vi "Get Relay Position.vi"(8 "error in (no error)":errorcluster, 10 "relay name":string, 11 "SLSC Switch in":refnum<class "SLSC Switch.lvclass">) -> (0 "error out":errorcluster, 2 "position":T1=10 items=["Open"=10, "Closed"=11], 3 "SLSC Switch out":refnum<class "SLSC Switch.lvclass">)   [LabVIEW 2015, in "SLSC Switch.lvlib" / "SLSC Switch.lvclass"]
doc: "Returns the relay position for the relay specified in relay name."
uses:
  SLSC Switch.lvclass
  Switch Action Processor/Switch Action Processor.lvclass
  Relay/Relay.lvclass
  slscsl/RelayPosition.ctl
  slscsl/slscsl.lvclass
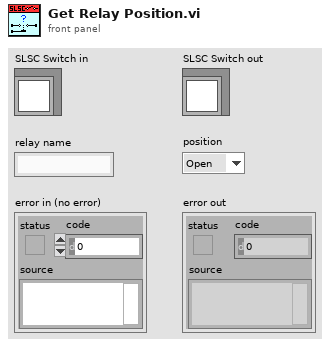
[diagram p1: front panel]
types:
  T1 = typedef "SLSC Switch.lvlib/slscsl.lvclass/RelayPosition.ctl" = i32
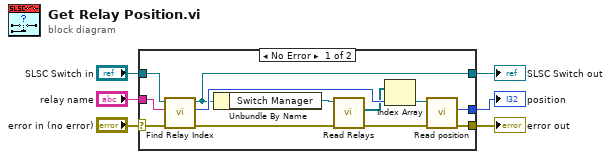
[diagram p0: block diagram]
diagram:
  n1 = case shown="No Error" "error in (no error)" {
    selector: "error in (no error)" -> [w17 w20]
    tunnel: [w7 w20] -> w5
    tunnel: "relay name" -> [w18 _]
    tunnel: [w16 _] -> w3
    tunnel: "SLSC Switch in" -> [w15 w19]
    tunnel: [w13 w19] -> w1
    frame No Error {
      n2 = call "Find Relay Index.vi"("error in (no error)"=w17, "relay string"=w18, "SLSC Switch in"=w15) -> ("error out"=w12:errorcluster, "index"=w14:i32, "SLSC Switch out"=w13:refnum<class "SLSC Switch.lvclass">)  [unwired: 6 in]
      n3 = Unbundle By Name(w13) -> ("Switch Manager"=w10:refnum<class "Switch Action Processor.lvclass">)
      n4 = call "Read Relays.vi"("error in (no error)"=w12, "Switch Action Processor in"=w10) -> ("error out"=w9:errorcluster, "Relays"=w11:refnum<class "Relay.lvclass">[])  [unwired: 8 in]
      n5 = Index Array(array=w11, index=w14) -> (element=w8:refnum<class "Relay.lvclass">)
      n6 = call "Read position.vi"("error in (no error)"=w9, "Relay in"=w8) -> ("error out"=w7:errorcluster, "position"=w16:T1)  [unwired: 7 in, 1 out]
    }
    frame Error {
    }
  }
  "error out" <- w5
  "position" <- w3
  "SLSC Switch out" <- w1
